vi "Update Image.vi"(0 "Image IN":T2, 2 "Scan Direction":T1 items=["Forward", "Reverse", "LineIn"], 7 "Image fraction IN":T2, 9 "Frame number":i32) -> (4 "Image ref OUT":T2)   [LabVIEW 2020]
uses:
  <vilib>/vision/Image Controls.llb/IMAQ Image.ctl
  VPD Controls/VPD Scan Direction.ctl
  Cameras/Camera Controls/Camera IMAQ Key Info.ctl
  <vilib>/vision/NI_Vision_Development_Module.lvlib
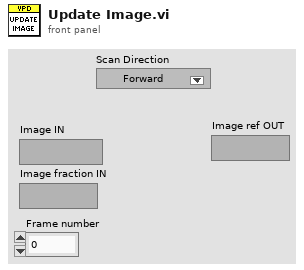
[diagram p1: front panel]
types:
  T1 = typedef "VPD Scan Direction.ctl" = i64
  T2 = typedef "IMAQ Image.ctl" = refnum<image>
  T3 = typedef "Camera IMAQ Key Info.ctl" = cluster{"Frame":u32, "Sensor Height":i32, "Sensor Width":i32, "ROI Height":i32, "ROI Width":i32, "ROI Enable?":bool, "Bit per Pixel":u8, "Binning factor":i32}
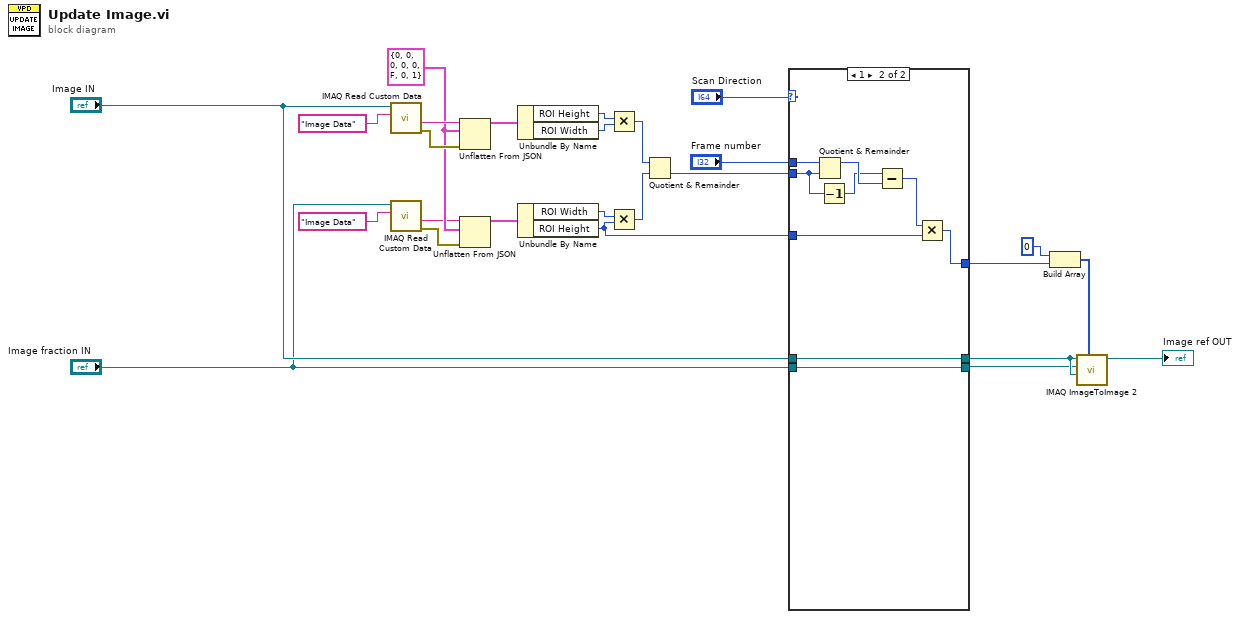
[diagram p0: block diagram]
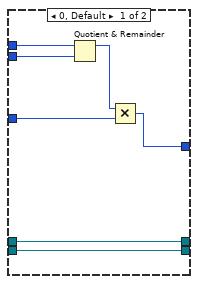
[diagram p2: hidden frame]
diagram:
  w22 = T3 {"Frame"=0, "Sensor Height"=0, "Sensor Width"=0, "ROI Height"=0, "ROI Width"=0, "ROI Enable?"=FALSE, "Bit per Pixel"=0, "Binning factor"=1} ("Camera IMAQ Key Info")
  n1 = call "IMAQ Read Custom Data"("Key"="Image Data", "Image"="Image IN") -> ("error out"=w24:errorcluster, "Custom Data Out"=w25:string)  [unwired: 7 in, 1 out]
  n2 = call "IMAQ Read Custom Data"("Key"="Image Data", "Image"="Image fraction IN") -> ("error out"=w21:errorcluster, "Custom Data Out"=w20:string)  [unwired: 7 in, 1 out]
  n3 = Unflatten From JSON(JSON string=w25, type and defaults=w22, error in (no error)=w24) -> (value=w23:T3)  [unwired: 4 in, 1 out]
  n4 = Unflatten From JSON(JSON string=w20, type and defaults=w22, error in (no error)=w21) -> (value=w19:T3)  [unwired: 4 in, 1 out]
  n5 = Unbundle By Name(w23) -> ("ROI Height"=w16:i32, "ROI Width"=w17:i32)
  n6 = Unbundle By Name(w19) -> ("ROI Width"=w15:i32, "ROI Height"=w6:i32)
  n7 = Multiply(x=w16, y=w17) -> (x*y=w14:i32)
  n8 = Multiply(x=w15, y=w6) -> (x*y=w13:i32)
  n9 = Quotient & Remainder(x=w14, y=w13) -> (floor(x/y)=w12:i32)  [unwired: 1 out]
  n10 = case shown="1" "Scan Direction" {
    tunnel: w12 -> [w33 w36]
    tunnel: "Frame number" -> [w32 w42]
    tunnel: [w30 w41] -> w8
    tunnel: w6 -> [w29 w40]
    tunnel: [w28 w37] -> w4
    tunnel: "Image IN" -> [w28 w37]
    tunnel: "Image fraction IN" -> [w27 w34]
    tunnel: [w27 w34] -> w1
    frame 0, Default {
      n11 = Quotient & Remainder(x=w32, y=w33) -> (x-y*floor(x/y)=w31:i32)  [unwired: 1 out]
      n12 = Multiply(x=w31, y=w29) -> (x*y=w30:i32)
    }
    frame 1 {
      n13 = Quotient & Remainder(x=w42, y=w36) -> (x-y*floor(x/y)=w39:i32)  [unwired: 1 out]
      n14 = Decrement(x=w36) -> (x-1=w35:i32)
      n15 = Subtract(x=w35, y=w39) -> (x-y=w38:i32)
      n16 = Multiply(x=w38, y=w40) -> (x*y=w41:i32)
    }
  }
  n17 = Build Array(0 ("element"), w8) -> (w10:i32[])
  n18 = call "IMAQ ImageToImage 2"("Offset Left/Top"=w10, "Image Dst"=w4, "Image Src (Small)"=w1, "Image Src (Large)"=w4) -> ("Image Dst Out"=→"Image ref OUT":T2)  [unwired: 6 in, 1 out]
